vi "Write merkers.vi"(0 "TCP Network Connection in":refnum<k5>, 1 "MW SCRITTURE":T1(array[cluster]), 2 "M REAL SCRITTURE (AO)":cluster{"MD":i16, "Descrizione":string}[](array[cluster]), 3 "AO (word)":dbl[](array[numeric]), 4 "AO (real) in":dbl[](array[numeric]), 5 "error in (no error)":errorcluster) -> (14 "TCP Network Connection out":refnum<k5>, 19 "error out":errorcluster)   [LabVIEW 2019]
uses:
  SIEMENS/S7Com_Source/S7Com_RW_CMD.ctl
  SIEMENS/S7Com_Source/S7Com_Address_Area.ctl
  SIEMENS/S7Com_Source/S7Com_Start_Add.ctl
  SIEMENS/S7Com_Source/S7Com_Transport_Size.ctl
  SIEMENS/S7Com_Source/S7Com_Function.ctl
  SIEMENS/S7Com_Source/S7Com_Data_Array.ctl
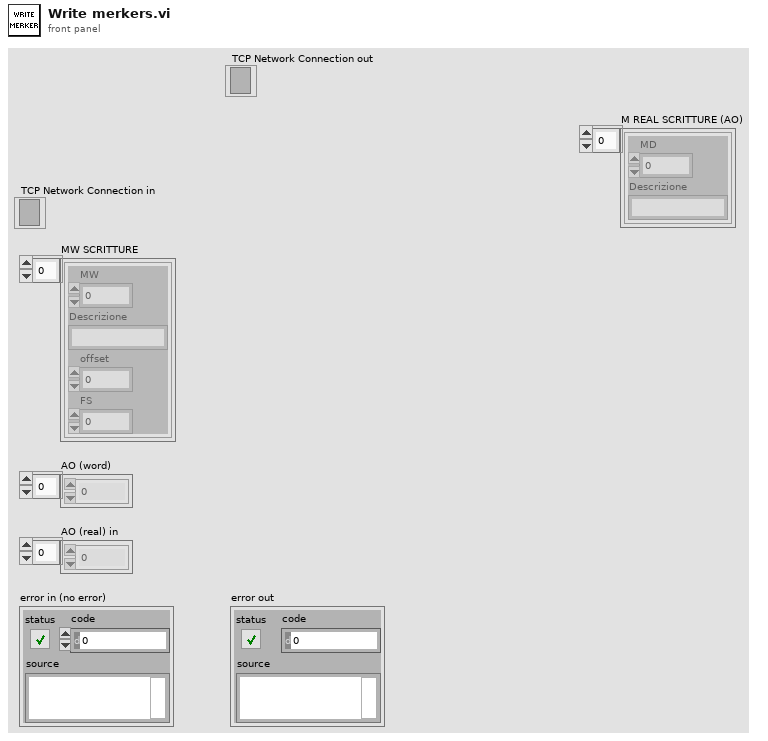
[diagram p1: front panel]
types:
  T1 = cluster{"MW":dbl, "Descrizione":string, "offset":dbl, "FS":dbl}[]
  T2 = typedef "S7Com_RW_CMD.ctl" = cluster{"Read Length":u16, "Data Block #":u16, "S7_Add_Area":T3, "Start Address":T4, "S7_Transport_Size":T5, "S7_Function":T6}
  T3 = typedef "S7Com_Address_Area.ctl" = u8
  T4 = typedef "S7Com_Start_Add.ctl" = u16
  T5 = typedef "S7Com_Transport_Size.ctl" = u8
  T6 = typedef "S7Com_Function.ctl" = u8
  T7 = typedef "S7Com_Data_Array.ctl" = i32[]
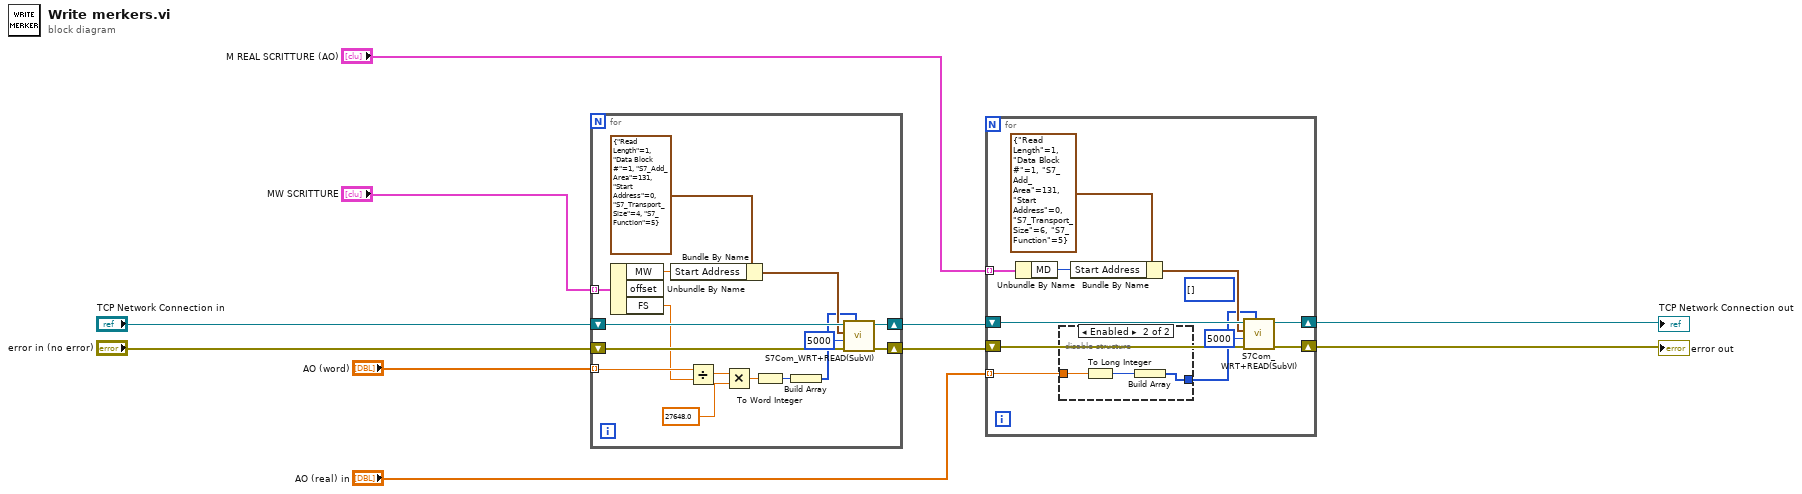
[diagram p0: block diagram]
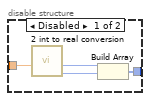
[diagram p2: hidden frame]
diagram:
  n1 = for {
    tunnel: "MW SCRITTURE" -> [w26] mode=indexing
    shift-right: [w20] -> w6
    shift-left: "error in (no error)" -> [w21]
    tunnel: "AO (word)" -> [w17] mode=indexing
    shift-right: [w22] -> w5
    shift-left: "TCP Network Connection in" -> [w23]
    n2 = Unbundle By Name(w26) -> ("MW"=w24:dbl, "FS"=w16:dbl)  [unwired: 1 out]
    n3 = Bundle By Name(cluster=T2 {"Read Length"=1, "Data Block #"=1, "S7_Add_Area"=131, "Start Address"=0, "S7_Transport_Size"=4, "S7_Function"=5} ("RW_CMD"), "Start Address"=w24) -> (w19:T2)
    n4 = Divide(x=w17, y=w16) -> (x/y=w15:dbl)
    n5 = Multiply(x=w15, y=27648.0) -> (x*y=w13:dbl)
    n6 = To Word Integer(number=w13) -> (16bit integer=w12:i16)
    n7 = Build Array(w12) -> (w18:i16[])
    n8 = call "S7Com_WRT+READ(SubVI).vi"("Write_Data"=w18, "error in"=w21, "timeout ms (25000)"=5000, "RW_CMD"=w19, "connection ID in"=w23) -> ("error out"=w20:errorcluster, "connection ID out"=w22:refnum<k5>)  [unwired: 2 out]
  }
  n9 = for {
    tunnel: "M REAL SCRITTURE (AO)" -> [w37] mode=indexing
    shift-right: [w31] -> w8
    shift-left: w6 -> [w32]
    shift-right: [w33] -> w7
    shift-left: w5 -> [w34]
    tunnel: "AO (real) in" -> [w27] mode=indexing
    (unwired) T7 [] ("Write_Data")
    n10 = Unbundle By Name(w37) -> ("MD"=w35:i16)
    n11 = disable-structure shown="Enabled" {
      disable-tunnel: [w39 w42] -> w28
      disable-tunnel: w27 -> [w38 w44]
      frame Disabled {
        n12 = call "2 int to real conversion.vi"("reale in"=w38) -> ("MW 15 0 out"=w40:i16, "MW 31 16 out"=w41:i16)  [unwired: 8 in, 1 out]
        n13 = Build Array(w41, w40) -> (w39:i16[])
      }
      frame Enabled {
        n14 = To Long Integer(number=w44) -> (32bit integer=w43:i32)
        n15 = Build Array(w43) -> (w42:i32[])
      }
    }
    n16 = Bundle By Name(cluster=T2 {"Read Length"=1, "Data Block #"=1, "S7_Add_Area"=131, "Start Address"=0, "S7_Transport_Size"=6, "S7_Function"=5} ("RW_CMD"), "Start Address"=w35) -> (w30:T2)
    n17 = call "S7Com_WRT+READ(SubVI).vi"("Write_Data"=w28, "error in"=w32, "timeout ms (25000)"=5000, "RW_CMD"=w30, "connection ID in"=w34) -> ("error out"=w31:errorcluster, "connection ID out"=w33:refnum<k5>)  [unwired: 2 out]
  }
  "error out" <- w8
  "TCP Network Connection out" <- w7
